vi "testper.vi"() -> ()   [LabVIEW 2012]
uses:
  <vilib>/DAQmx/read.llb/DAQmx Read (Analog 2D DBL NChan NSamp).vi
  <vilib>/DAQmx/write.llb/DAQmx Write (Analog DBL 1Chan 1Samp).vi
panel:
  in  "Stoppspänning":dbl
  in  "Startspänning":dbl
  in  "Antal punkter":i32
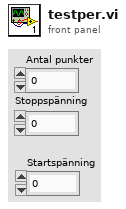
[diagram p1: front panel]
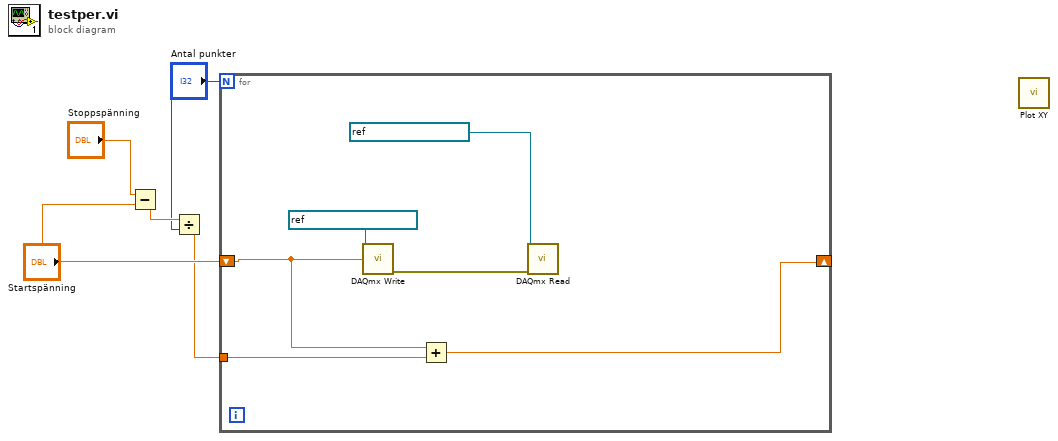
[diagram p0: block diagram]
diagram:
  n1 = Subtract(x="Stoppspänning", y="Startspänning") -> (x-y=w3:dbl)
  n2 = Divide(x=w3, y="Antal punkter") -> (x/y=w1:dbl)
  n3 = for {
    N: "Antal punkter" -> [_]
    shift-right: [w6] -> _
    shift-left: "Startspänning" -> [w8]
    tunnel: w1 -> [w7]
    n4 = call-poly <vilib>:"DAQmx Write.vi"("task/channels in"=refnum<k21> "MyVoltageOutTask", "data"=w8) -> ("error out"=w9:errorcluster)  [unwired: 11 in, 2 out]
    n5 = Add(x=w8, y=w7) -> (x+y=w6:dbl)
    n6 = call-poly <vilib>:"DAQmx Read.vi"("task/channels in"=refnum<k21> "MyVoltageTask_3", "error in"=w9) -> ()  [unwired: 11 in, 3 out]
  }
  n7 = call <vilib>:"Plot XY.vi"() -> ()  [unwired: 15 in, 1 out]
